vi "All Complex.vi"() -> (3 "GEMM Benchmark":cluster{i32[], dbl[]}[](graph))   [LabVIEW 2020]
doc: "Execute GEMM Process for different size on different Toolkits (Accelerator/Culab/CUDA/LabVIEW/G2CPU) and LabVIEW(CPU)."
uses:
  <vilib>/Natan Biesmans/G2CPU GPU and CPU HPC Toolkit/ArrayFire Driver/TypeDefs/backend.ctl
  <vilib>/Natan Biesmans/G2CPU GPU and CPU HPC Toolkit/ArrayFire Driver/AF.lvlib
panel:
  out "Accelerator DirectML":bool
  out "Accelerator CUDA":bool
  out "Culab":bool
  out "Accelerator TRT":bool
  out "LabVIEW":bool
  out "G2CPU":bool
  out "G2CPU Time":dbl
  out "LabVIEW Time":dbl
  out "Accelerator CUDA Time":dbl
  out "Culab Time":dbl
  out "Accelerator TRT Time":dbl
  # "Complex Process"
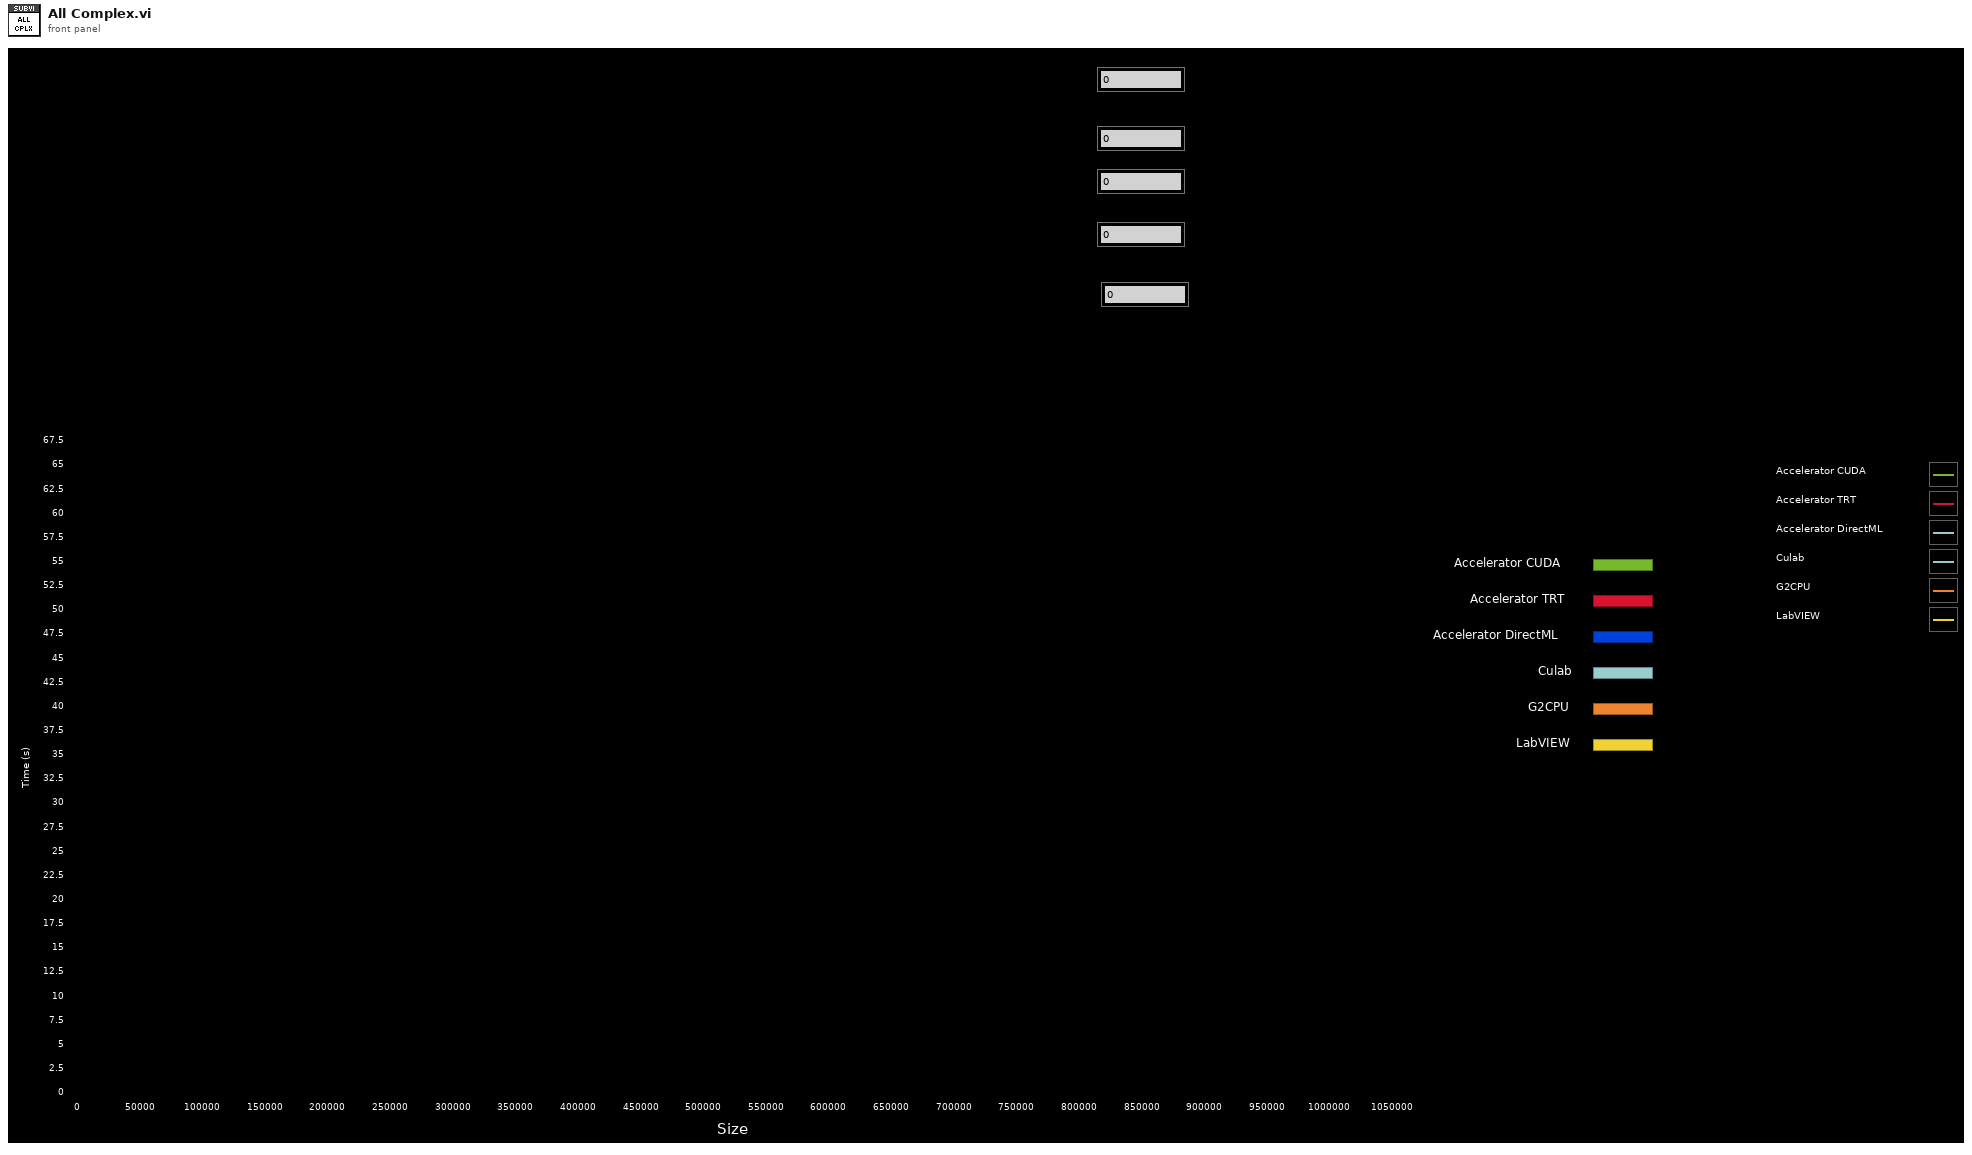
[diagram p1: front panel]
types:
  T1 = cluster{"intra_op_num_threads":i32, "inter_op_num_threads":i32, "execution_mode":enum16{"ORT_SEQUENTIAL", "ORT_PARALLEL"}, "deterministic_compute":bool, "graph_optimization_level":u16, "optimized_model_file_path":path, "profiling output dir":path}
  T2 = typedef "AF.lvlib/backend.ctl" = u32
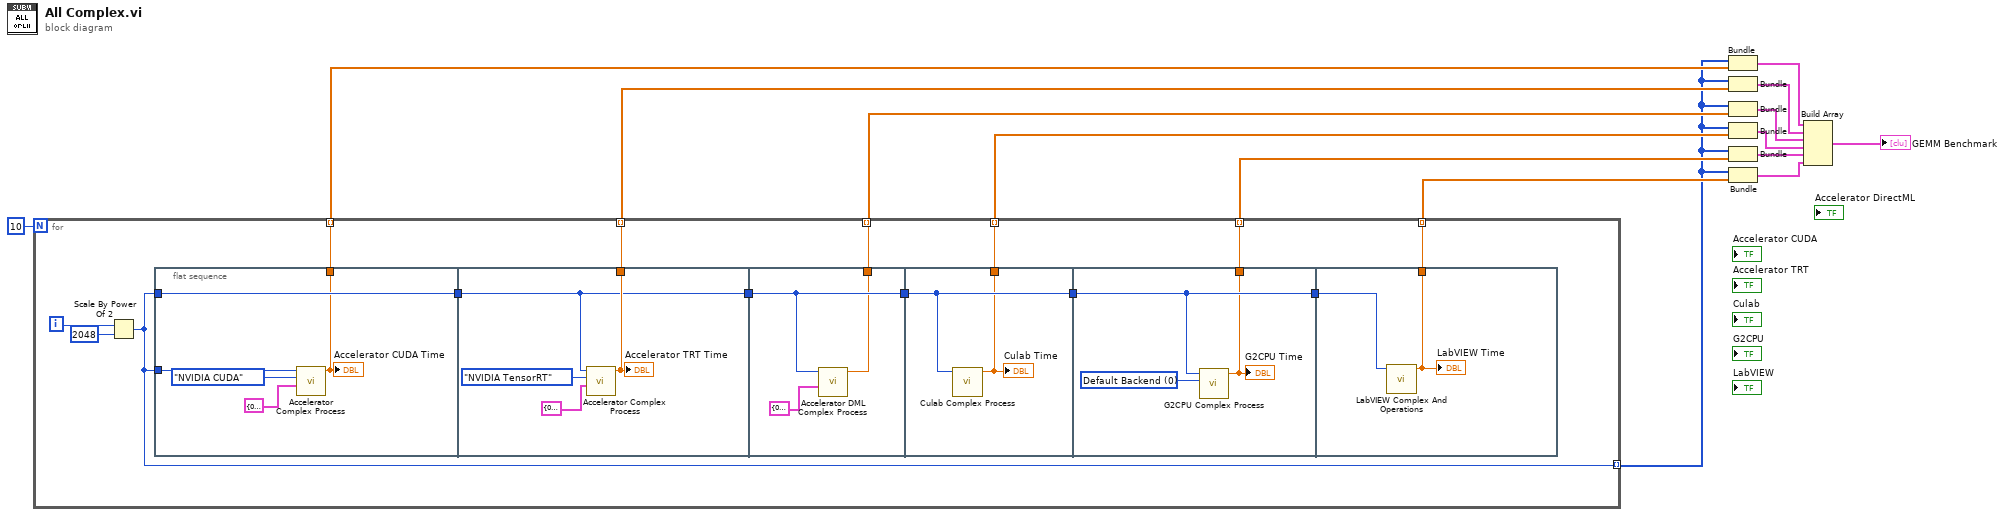
[diagram p0: block diagram]
diagram:
  n1 = for {
    N: 10 -> [_]
    tunnel: [w29] -> w14 mode=indexing
    tunnel: [w28] -> w13 mode=indexing
    tunnel: [w25] -> w1 mode=indexing
    tunnel: [w23] -> w7 mode=indexing
    tunnel: [w21] -> w9 mode=indexing
    tunnel: [w19] -> w6 mode=indexing
    tunnel: [w16] -> w2 mode=indexing
    i -> [w26]
    n2 = Scale By Power Of 2(n=w26, x=2048) -> (x*2^n=w25:i32)
    n3 = flat-sequence {
      tunnel: w25 -> [w34]
      tunnel: w25 -> [w33]
      tunnel: [w34] -> w22
      tunnel: [w32] -> w21
      tunnel: [w37] -> w18
      tunnel: [w38] -> w29
      tunnel: w22 -> [w37]
      tunnel: w18 -> [w41]
      tunnel: [w41] -> w17
      tunnel: [w39] -> w16
      tunnel: w17 -> [w43]
      tunnel: [w43] -> w20
      tunnel: [w42] -> w28
      tunnel: w20 -> [w46]
      tunnel: [w46] -> w24
      tunnel: [w45] -> w19
      tunnel: w24 -> [w47]
      tunnel: [w48] -> w23
      frame #0 {
        n4 = call "Accelerator Complex Process.vi"("Sessions Parameters"=T1 {"intra_op_num_threads"=0, "inter_op_num_threads"=0, "execution_mode"=enum."ORT_SEQUENTIAL", "deterministic_compute"=FALSE, "graph_optimization_level"=1, "optimized_model_file_path"=path "", "profiling output dir"=path ""}, "Execution Device"=enum16{"CPU", "NVIDIA CUDA", "NVIDIA TensorRT"}."NVIDIA CUDA", "X size"=w33) -> ("Accelerator Time"=w32:dbl)  [unwired: 8 in]
        "Accelerator CUDA Time" <- w32
      }
      frame #1 {
        n5 = call "Accelerator Complex Process.vi"("Sessions Parameters"=T1 {"intra_op_num_threads"=0, "inter_op_num_threads"=0, "execution_mode"=enum."ORT_SEQUENTIAL", "deterministic_compute"=FALSE, "graph_optimization_level"=1, "optimized_model_file_path"=path "", "profiling output dir"=path ""}, "Execution Device"=enum16{"CPU", "NVIDIA CUDA", "NVIDIA TensorRT"}."NVIDIA TensorRT", "X size"=w37) -> ("Accelerator Time"=w38:dbl)  [unwired: 8 in]
        "Accelerator TRT Time" <- w38
      }
      frame #2 {
        n6 = call "Accelerator DML Complex Process.vi"("Sessions Parameters"=T1 {"intra_op_num_threads"=0, "inter_op_num_threads"=0, "execution_mode"=enum."ORT_SEQUENTIAL", "deterministic_compute"=FALSE, "graph_optimization_level"=1, "optimized_model_file_path"=path "", "profiling output dir"=path ""}, "X size"=w41) -> ("Accelerator Time"=w39:dbl)  [unwired: 9 in]
      }
      frame #3 {
        n7 = call "Culab Complex Process.vi"("X size"=w43) -> ("Culab Time"=w42:dbl)  [unwired: 10 in]
        "Culab Time" <- w42
      }
      frame #4 {
        w44 = T2 0 items=["Default Backend"=0, "CPU Backend"=1, "CUDA Backend"=2, "OPENCL Backend"=4, "Intel OneAPI Backend"=8] ("Backend")
        n8 = call "G2CPU Complex Process.vi"("Backend"=w44, "X size"=w46) -> ("G2CPU Time"=w45:dbl)  [unwired: 9 in]
        "G2CPU Time" <- w45
      }
      frame #5 {
        n9 = call "LabVIEW Complex And Operations.vi"("X size"=w47) -> ("LabVIEW Time"=w48:dbl)  [unwired: 10 in]
        "LabVIEW Time" <- w48
      }
    }
  }
  n10 = Bundle(w1, w9) -> (w10:cluster{i32[], dbl[]})  [unwired: 1 in]
  n11 = Bundle(w1, w14) -> (w11:cluster{i32[], dbl[]})  [unwired: 1 in]
  n12 = Bundle(w1, w2) -> (w3:cluster{i32[], dbl[]})  [unwired: 1 in]
  n13 = Bundle(w1, w13) -> (w4:cluster{i32[], dbl[]})  [unwired: 1 in]
  n14 = Bundle(w1, w6) -> (w8:cluster{i32[], dbl[]})  [unwired: 1 in]
  n15 = Bundle(w1, w7) -> (w5:cluster{i32[], dbl[]})  [unwired: 1 in]
  n16 = Build Array(w10, w11, w3, w4, w8, w5) -> (→"GEMM Benchmark":cluster{i32[], dbl[]}[])
